vi "ODE Simulation Parameters.vi"(4 "Simulation Parameters In":T1={"Initial Time"=0.0, "Final Time"=100.0, "Time Step"=0.1, "Absolute Tolerance"=0.001, "Relative Tolerance"=1e-06, "Type of Continuous Solver"=enum."Runge-Kutta 45 (variable)", "Discrete Time Step"=2.0, "Minimum Time Step"=1e-06, "Maximum Time Step"=1.0, "Initial Time Step"=0.1} {"Initial Time Step" min=0.0; "Maximum Time Step" min=0.0; "Minimum Time Step" min=0.0; "Discrete Time Step" min=0.0; "Relative Tolerance" min=0.0; "Absolute Tolerance" min=0.0; "Time Step" min=0.0}) -> (0 "Status":string, 1 "Simulation Parameters Out":T1={"Initial Time"=0.0, "Final Time"=100.0, "Time Step"=0.1, "Absolute Tolerance"=0.001, "Relative Tolerance"=1e-06, "Type of Continuous Solver"=enum."Runge-Kutta 45 (variable)", "Discrete Time Step"=2.0, "Minimum Time Step"=1e-06, "Maximum Time Step"=1.0, "Initial Time Step"=0.1} {"Initial Time Step" min=0.0; "Maximum Time Step" min=0.0; "Minimum Time Step" min=0.0; "Discrete Time Step" min=0.0; "Relative Tolerance" min=0.0; "Absolute Tolerance" min=0.0; "Time Step" min=0.0})   [LabVIEW 2014]
uses:
  ODE Simulation Parameters.ctl
  <vilib>/Simulation/Implementation/Shared/SIM Continuous Solvers.ctl
panel:
  in  "Cancel Button":bool
  in  "OK Button":bool
  in  "Simulation Parameters":T1={"Initial Time"=0.0, "Final Time"=20.0, "Time Step"=0.1, "Absolute Tolerance"=0.001, "Relative Tolerance"=1e-06, "Type of Continuous Solver"=enum."Runge-Kutta 45 (variable)", "Discrete Time Step"=2.0, "Minimum Time Step"=1e-06, "Maximum Time Step"=1.0, "Initial Time Step"=0.1} {"Initial Time Step" min=0.0; "Maximum Time Step" min=0.0; "Minimum Time Step" min=0.0; "Discrete Time Step" min=0.0; "Relative Tolerance" min=0.0; "Absolute Tolerance" min=0.0; "Time Step" min=0.0}
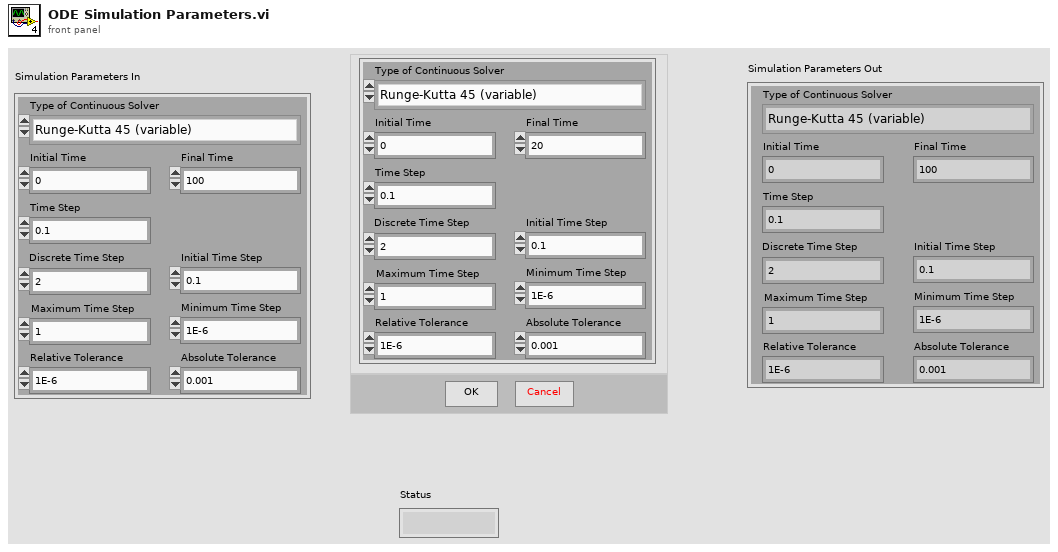
[diagram p1: front panel]
types:
  T1 = typedef "ODE Simulation Parameters.ctl" = cluster{"Initial Time":dbl, "Final Time":dbl, "Time Step":dbl, "Absolute Tolerance":dbl, "Relative Tolerance":dbl, "Type of Continuous Solver":T2, "Discrete Time Step":dbl, "Minimum Time Step":dbl, "Maximum Time Step":dbl, "Initial Time Step":dbl}
  T2 = typedef "SIM Continuous Solvers.ctl" = enum16{"Runge-Kutta 1 (Euler)", "Runge-Kutta 2", "Runge-Kutta 3", "Runge-Kutta 4", "Runge-Kutta 23 (variable)", "Runge-Kutta 45 (variable)", "BDF (variable)", "Adams-Moulton (variable)", "Rosenbrock (variable)", "Discrete States Only"}
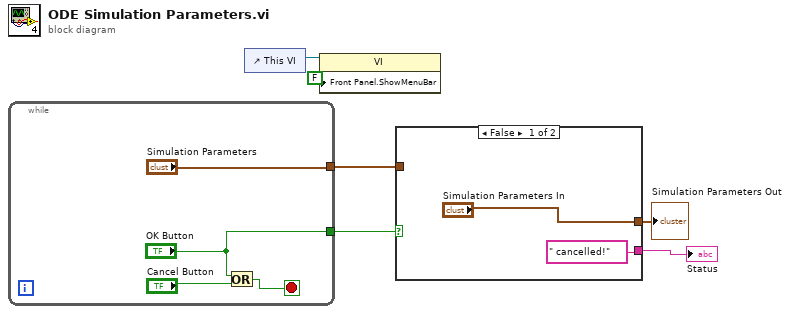
[diagram p0: block diagram]
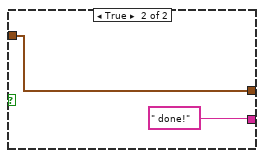
[diagram p2: hidden frame]
diagram:
  n1 = while {
    tunnel: ["Simulation Parameters"] -> w5
    tunnel: ["OK Button"] -> w6
    stop <- w9 stop-if-true
    n2 = Or(x="OK Button", y="Cancel Button") -> (x .or. y?=w9:bool)
  }
  n3 = control-ref of="This VI"() -> (w3:refnum<vi>)
  n4 = property class="VI"(reference=w3, "Front Panel.ShowMenuBar"=FALSE ("Front Panel Window:Show Menu Bar")) -> ()  [unwired: 1 in, 2 out]
  n5 = case shown="False" w6 {
    tunnel: w5 -> [_ w14]
    tunnel: ["Simulation Parameters In" w14] -> w1
    tunnel: [" cancelled!" " done!"] -> w4
    frame False {
    }
    frame True {
    }
  }
  "Status" <- w4
  "Simulation Parameters Out" <- w1
